vi "Set TDMS Group Names.vi"(10 "Group Names":string[](array[string]), 11 "App Data In":T1) -> (3 "App Data Out":T1)   [LabVIEW 2019]
uses:
  TypeDef/App Data.ctl
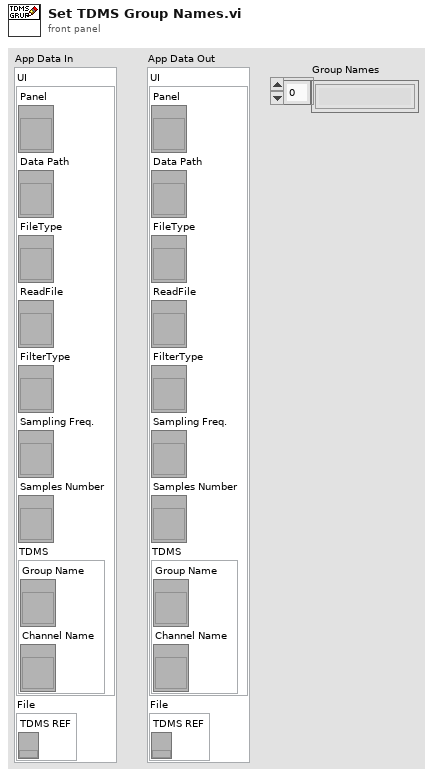
[diagram p1: front panel]
types:
  T1 = typedef "App Data.ctl" = cluster{"UI":cluster{"Panel":refnum<vi>, "Data Path":refnum<vi>, "FileType":refnum<vi>, "ReadFile":refnum<vi>, "FilterType":refnum<vi>, "Sampling Freq.":refnum<vi>, "Samples Number":refnum<vi>, "TDMS":cluster{"Group Name":refnum<vi>, "Channel Name":refnum<vi>}}, "File":cluster{"TDMS REF":refnum<k34>}}
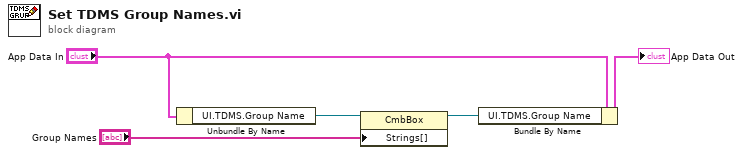
[diagram p0: block diagram]
diagram:
  n1 = Unbundle By Name("App Data In") -> ("UI.TDMS.Group Name"=w4:refnum<vi>)
  n2 = property class="CmbBox"(reference=w4, "Strings[]"="Group Names") -> (reference out=w5:refnum<vi>)  [unwired: 1 in, 1 out]
  n3 = Bundle By Name(cluster="App Data In", "UI.TDMS.Group Name"=w5) -> (→"App Data Out":T1)
